vi "Square with Sign.vi"(11 "Turret Setpoint":dbl) -> (3 "Numeric":dbl)   [LabVIEW 2018]
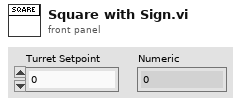
[diagram p1: front panel]
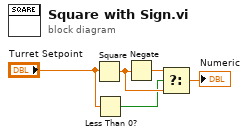
[diagram p0: block diagram]
diagram:
  n1 = Square(x="Turret Setpoint") -> (x^2=w3:dbl)
  n2 = Less Than 0?(x="Turret Setpoint") -> (x < 0?=w1:bool)
  n3 = Negate(x=w3) -> (-x=w4:dbl)
  n4 = Select(t=w4, s=w1, f=w3) -> (s? t:f=→"Numeric":dbl)
